vi "TEST TRANSFER.vi"() -> ()   [LabVIEW 2016]
uses:
  <vilib>/visionFPGA/Controls/IMAQ FPGA Pixel Bus u8x1.ctl
  <vilib>/rvi/Emulation/niFpgaSctlEmulationGetInTimedLoop.vi
  <vilib>/rvi/Emulation/niFpgaProcessEmulError.vi
  <vilib>/rvi/Emulation/niFpgaGetClockAttributes.vi
  <vilib>/rvi/Emulation/niFpgaEmulationReportErrorSimple.vi
  <vilib>/rvi/interface/RandomDataEmulation/niFpgaRandomDataHandleErrors.vi
  <vilib>/visionFPGA/Basics/Pixel Bus to FIFO/IMAQ FPGA Pixel Bus to FIFO U8x1.vi
  <vilib>/rvi/Emulation/niFpgaCriticalErrorInLSC.vi
  <vilib>/rvi/DataTransferAndStorage/Container/XNode/niFpgaContainer.xnode
  <vilib>/rvi/interface/RandomDataEmulation/nirviRandomDataFpgaReadWriteTemplate.vi
  <vilib>/visionFPGA/NI_VDM_FPGA_Basics.lvlib
panel:
  out "Numeric":u32
  in  "Pixel Bus In":T1
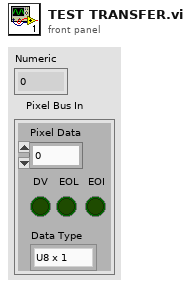
[diagram p1: front panel]
types:
  T1 = typedef "IMAQ FPGA Pixel Bus u8x1.ctl" = cluster{"Pixel Data":u8, "DV":bool, "EOL":bool, "EOI":bool, "Data Type":enum16{"U8 x 1"}}
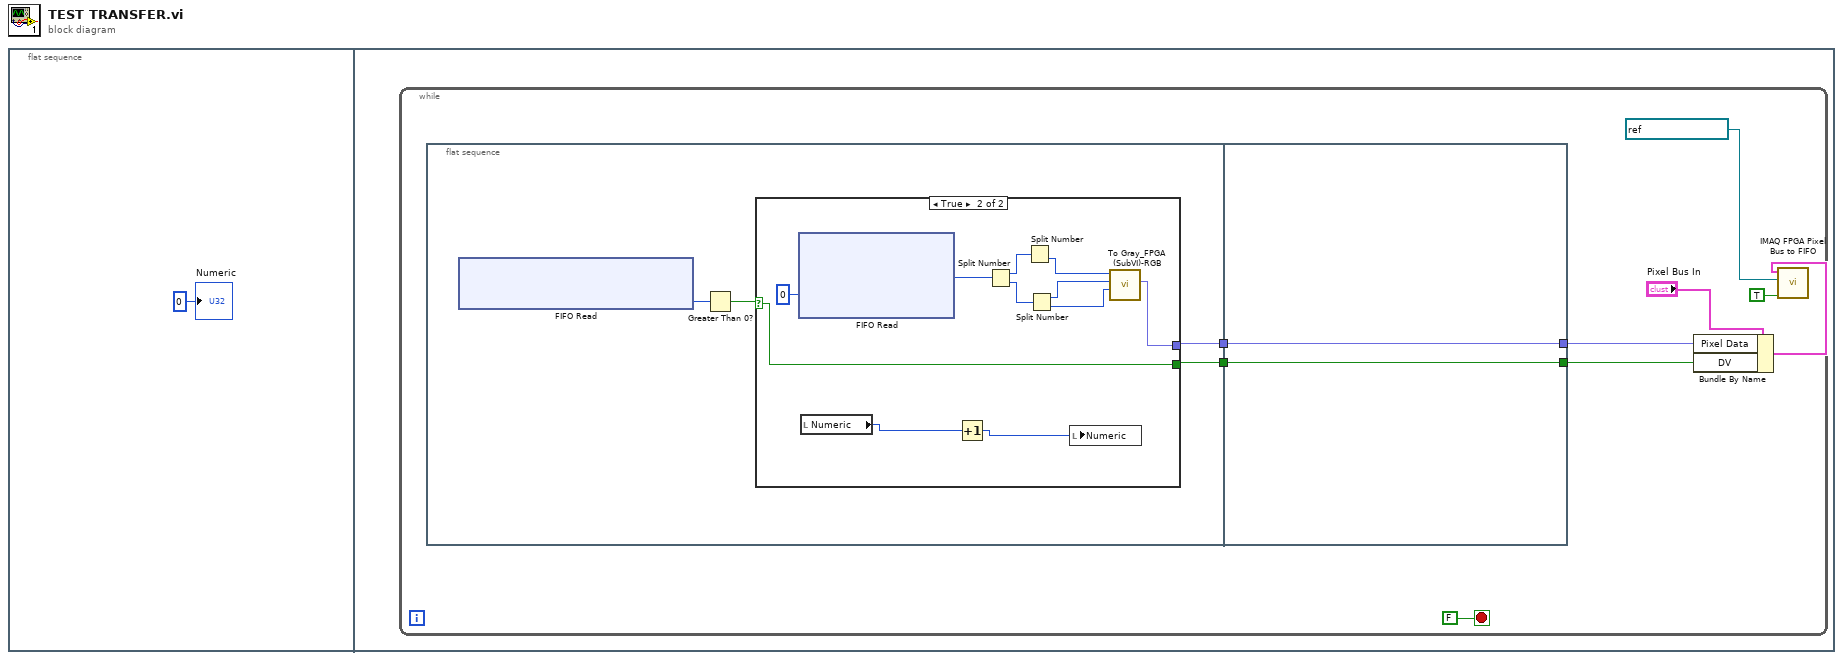
[diagram p0: block diagram]
diagram:
  n1 = flat-sequence {
    frame #0 {
      "Numeric" <- i16 0
    }
    frame #1 {
      n2 = while {
        stop <- FALSE stop-if-true
        n3 = flat-sequence {
          tunnel: [w12] -> w3
          tunnel: [w11] -> w2
          tunnel: [w27] -> w4
          tunnel: [w28] -> w6
          tunnel: w3 -> [w28]
          tunnel: w2 -> [w27]
          frame #0 {
            n4 = xnode "FIFO Read"() -> ("Number of Elements to Read"=w14:u32)  [unwired: 1 in, 1 out]
            n5 = Greater Than 0?(x=w14) -> (x > 0?=w13:bool)
            n6 = case shown="True" w13 {
              selector: w13 -> [w15 w18]
              tunnel: [_ w19] -> w12
              tunnel: [w15 w18] -> w11
              frame False {
              }
              frame True {
                n7 = xnode "FIFO Read"("Timeout"=0) -> ("Element"=w26:u32)  [unwired: 1 in, 2 out]
                n8 = local read "Numeric"() -> (w17:u32)
                n9 = Increment(x=w17) -> (x+1=w16:u32)
                n10 = Split Number(x=w26) -> (hi(x)=w24:u16, lo(x)=w25:u16)
                n11 = Split Number(x=w24) -> (lo(x)=w23:u8)  [unwired: 1 out]
                n12 = Split Number(x=w25) -> (hi(x)=w22:u8, lo(x)=w21:u8)
                n13 = local write "Numeric"(w16) -> ()
                n14 = call "To Gray_FPGA (SubVI)-RGB.vi"("B"=w21, "G"=w22, "R"=w23) -> ("Data Out"=w19:fxp<+,8,8>)  [unwired: 8 in]
              }
            }
          }
          frame #1 {
          }
        }
        n15 = Bundle By Name(cluster="Pixel Bus In", "Pixel Data"=w6, "DV"=w4) -> (w8:T1)
        n16 = call-poly <vilib>:"IMAQ FPGA Pixel Bus to FIFO.vi"("Input Valid"=TRUE, "Destination Image FIFO"=refnum<k21> "Gaussian 1-1", "Pixel Bus In"=w8) -> ()  [unwired: 8 in, 1 out]
      }
    }
  }
